vi "fix db location.vi"(8 "error in (no error)":errorcluster) -> (0 "error out":errorcluster, 3 "BP Array":T1[](array[typedef]) {"File Location" items=["Mars Data Processing Factility"=-1, "Local Cache "=0, "Storage"=1]})   [LabVIEW 2011]
uses:
  C:/Users/Clavius/Desktop/LabView VIs/Database2.0/Batch Processor/bp_cluster.ctl
  C:/Users/Clavius/Desktop/LabView VIs/Database2.0/Private/File_location.ctl
  <vilib>/addons/database/Auxilliary.llb/DB Tools Cursor Type.ctl
  <vilib>/addons/database/Connection.llb/Conn Execute.vi
  <vilib>/addons/database/Recordset.llb/Rec Fetch Recordset Data (R).vi
  <vilib>/addons/database/Recordset.llb/Rec Destroy - Connection.vi
  <vilib>/addons/database/_DB Variant To Data/Database Variant To Data.xnode
  <vilib>/addons/database/NI_Database_API.lvlib
panel:
  in  "Time Stamp":timestamp
  out "size(s)":i32
  out "SQL Query Sintax":string
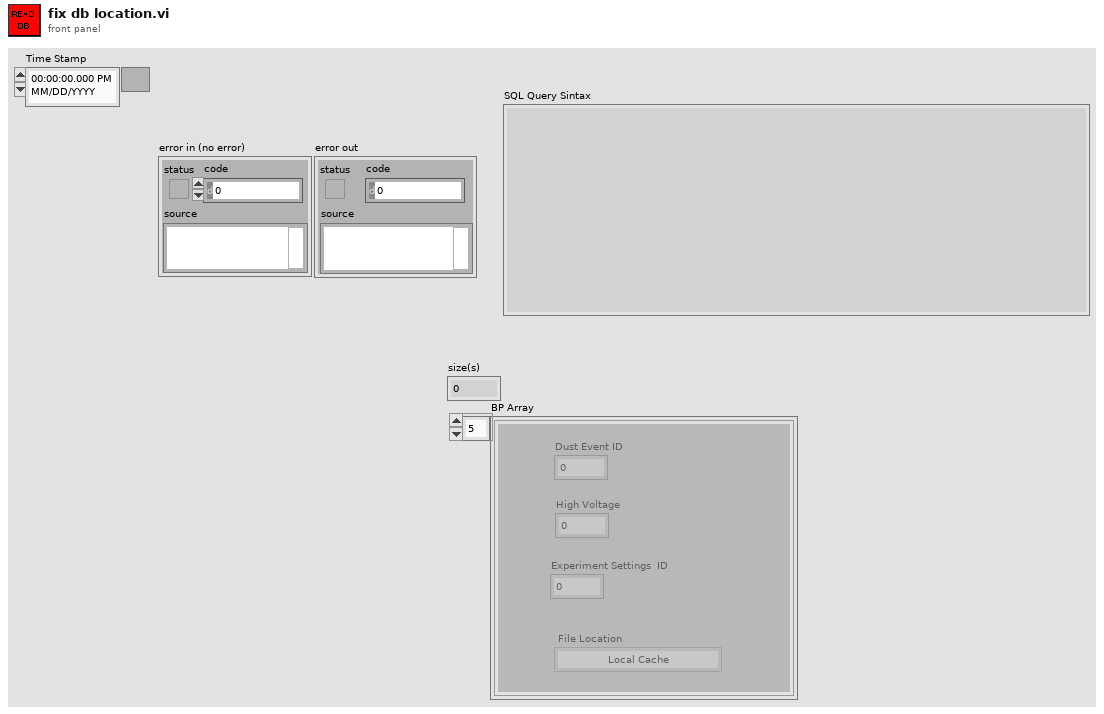
[diagram p1: front panel]
types:
  T1 = typedef "bp_cluster.ctl" = cluster{"Dust Event ID":i64, "High Voltage":sgl, "Experiment Settings  ID":i64, "File Location":T2}
  T2 = typedef "File_location.ctl" = i8
  T3 = typedef "NI_Database_API.lvlib/DB Tools Cursor Type.ctl" = enum16{"forward-only", "keyset", "dynamic", "static"}
  T4 = typedef "NI_Database_API.lvlib/Conn ObjectReference.ctl" = refnum<k1>
  T5 = typedef "NI_Database_API.lvlib/Rec ObjectReference.ctl" = refnum<k1>
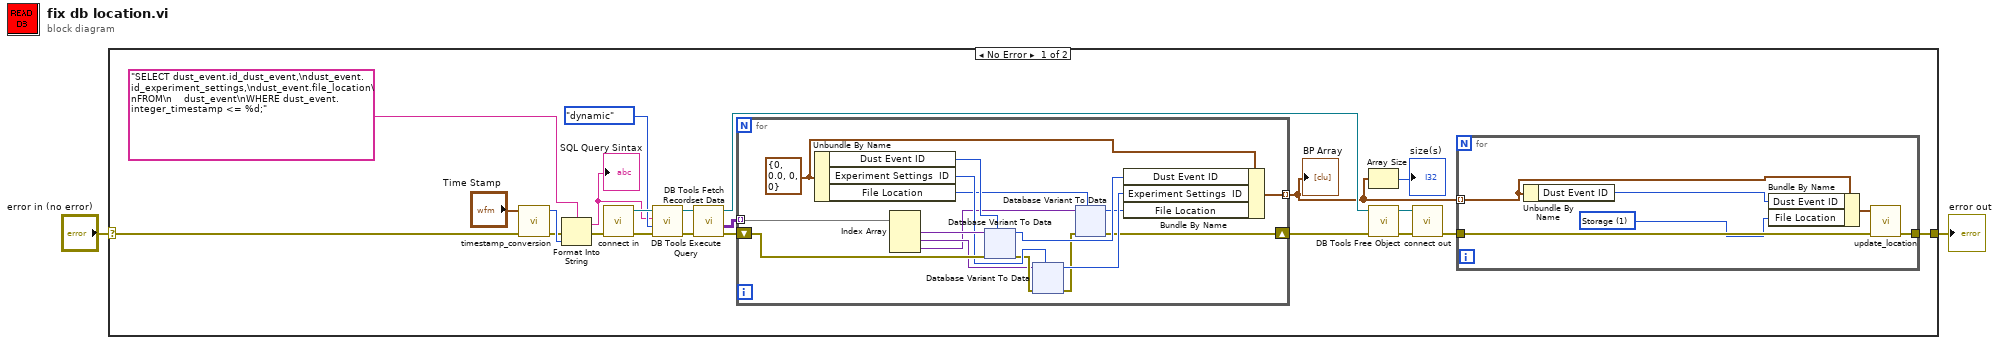
[diagram p0: block diagram]
diagram:
  n1 = case shown="No Error" "error in (no error)" {
    selector: "error in (no error)" -> [w7 w143]
    tunnel: [w3 w143] -> w1
    frame No Error {
      n2 = call "timestamp_conversion.vi"("error in (no error)"=w7, "Time Stamp"="Time Stamp") -> ("error out"=w8:errorcluster, "Integer Time"=w10:i64)  [unwired: 7 in]
      n3 = Format Into String(format string="SELECT dust_event.id_dust_event,\ndust_event.id_experiment_settings,\ndust_event.file_location\nFROM\n    dust_event\nWHERE dust_event.integer_timestamp <= %d;" ("string"), error in=w8, w10) -> (resulting string=w11:string, error out=w6:errorcluster)  [unwired: 1 in]
      "SQL Query Sintax" <- w11
      n4 = call "connect in.vi"("error in (no error)"=w6) -> ("error out"=w18:errorcluster, "Database Connection"=w19:T4)  [unwired: 6 in, 1 out]
      n5 = call-poly <vilib>:"DB Tools Execute Query.vi"("error in (no error)"=w18, "cursor type"=DB_Tools_Cursor_Type."dynamic", "SQL query"=w11, "connection reference"=w19) -> ("error out"=w23:errorcluster, "recordset reference"=w24:T5)  [unwired: 4 in]
      n6 = call-poly <vilib>:"DB Tools Fetch Recordset Data.vi"("error in (no error)"=w23, "recordset reference"=w24) -> ("error out"=w21:errorcluster, "recordset data"=w16:variant[][], "recordset reference out"=w22:T5)  [unwired: 3 in]
      n7 = for {
        tunnel: w16 -> [w46] mode=indexing
        shift-right: [w31] -> w20
        shift-left: w21 -> [w45]
        tunnel: [w43] -> w5 mode=indexing
        w40 = T1 {"Dust Event ID"=0, "High Voltage"=0.0, "Experiment Settings  ID"=0, "File Location"=0} ("Batch Processing Cluster")
        n8 = Unbundle By Name(w40) -> ("Dust Event ID"=w42:i64, "Experiment Settings  ID"=w39:i64, "File Location"=w34:T2)
        n9 = Index Array(array=w46) -> (element #1=w44:variant, element #2=w36:variant, element #3=w35:variant)  [unwired: 3 in]
        n10 = xnode "Database Variant To Data"("database variant"=w44, "error in"=w45, "type"=w42) -> ("data"=w41:i64, "error out"=w37:errorcluster)
        n11 = xnode "Database Variant To Data"("database variant"=w36, "error in"=w37, "type"=w39) -> ("data"=w38:i64, "error out"=w32:errorcluster)
        n12 = xnode "Database Variant To Data"("database variant"=w35, "error in"=w32, "type"=w34) -> ("data"=w33:T2, "error out"=w31:errorcluster)
        n13 = Bundle By Name(cluster=w40, "Dust Event ID"=w41, "Experiment Settings  ID"=w38, "File Location"=w33) -> (w43:T1)
      }
      "BP Array" <- w5
      n14 = Array Size(array=w5) -> (size(s)=→"size(s)":i32)
      n15 = call-poly <vilib>:"DB Tools Free Object.vi"("error in (no error)"=w20, "recordset reference"=w22) -> ("error out"=w14:errorcluster, "connection reference"=w17:T4)  [unwired: 8 in]
      n16 = call "connect out.vi"("error in (no error)"=w14, "connection reference"=w17) -> ("error out"=w4:errorcluster)  [unwired: 9 in]
      n17 = for {
        tunnel: w5 -> [w28] mode=indexing
        tunnel: w4 -> [w30]
        tunnel: [w29] -> w3
        w25 = T2 1 items=["Mars Data Processing Factility"=-1, "Local Cache "=0, "Storage"=1] ("File Location")
        n18 = Unbundle By Name(w28) -> ("Dust Event ID"=w27:i64)
        n19 = Bundle By Name(cluster=w28, "Dust Event ID"=w27, "File Location"=w25) -> (w26:T1)
        n20 = call "update_location.vi"("error in (no error)"=w30, "Batch Processing Cluster"=w26) -> ("error out"=w29:errorcluster)  [unwired: 8 in, 1 out]
      }
    }
    frame Error {
    }
  }
  "error out" <- w1
